vi "pruebas.vi"(11 "Image":T1) -> ()   [LabVIEW 2020]
uses:
  <vilib>/vision/Image Controls.llb/IMAQ Image.ctl
  <vilib>/picture/picture.llb/Draw True-Color Pixmap.vi
  <vilib>/Analysis/NI_AALBase.lvlib
panel:
  in  "alfa":dbl(slide) scale=0.0..5.0
  in  "S":dbl=30.0 format="%#_13g"
  in  "V":dbl=20.0 format="%#_13g"
  in  "Tamaño de máscara":i32
  out "Color":u32(colorbox)
  out "2D Picture":picture
  in  "Factor diezmado":i32=60
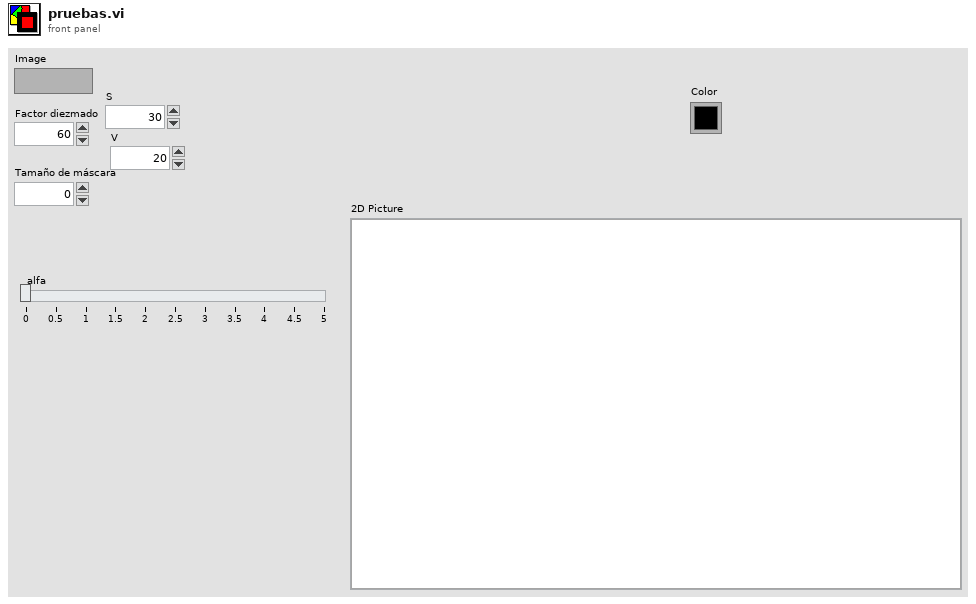
[diagram p1: front panel]
types:
  T1 = typedef "IMAQ Image.ctl" = refnum<image>
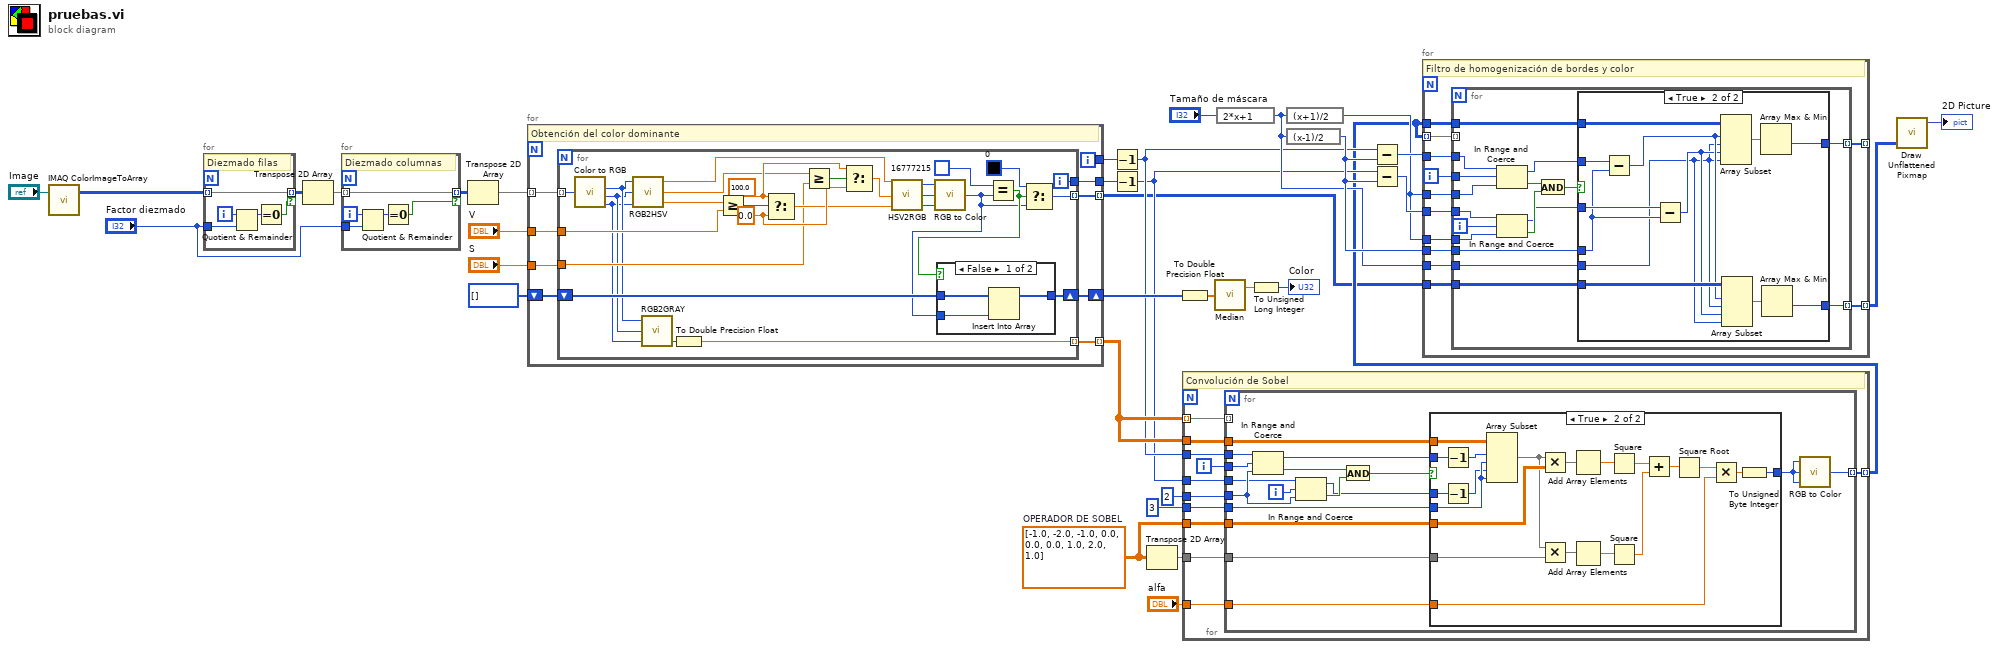
[diagram p0: block diagram]
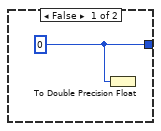
[diagram p2: hidden frame]
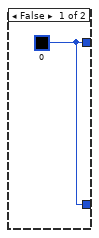
[diagram p3: hidden frame]
diagram:
  w5 = dbl[][] [[-1.0, -2.0, -1.0], [0.0, 0.0, 0.0], [1.0, 2.0, 1.0]]  # OPERADOR DE SOBEL
  n1 = call "IMAQ ColorImageToArray"("Image"="Image") -> ("Image Pixels (U32)"=w31:u32[][])  [unwired: 3 in, 2 out]
  n2 = for {
    tunnel: w31 -> [w39] mode=indexing
    tunnel: [w39] -> w34 mode=indexing if=w36
    tunnel: "Factor diezmado" -> [w35]
    i -> [w38]
    # "Diezmado filas"
    n3 = Quotient & Remainder(x=w38, y=w35) -> (x-y*floor(x/y)=w37:i32)  [unwired: 1 out]
    n4 = Equal To 0?(x=w37) -> (x = 0?=w36:bool)
  }
  n5 = Transpose 2D Array(2D array=w34) -> (transposed array=w33:u32[][])
  n6 = for {
    tunnel: w33 -> [w44] mode=indexing
    tunnel: [w44] -> w30 mode=indexing if=w41
    tunnel: "Factor diezmado" -> [w40]
    i -> [w43]
    # "Diezmado columnas"
    n7 = Quotient & Remainder(x=w43, y=w40) -> (x-y*floor(x/y)=w42:i32)  [unwired: 1 out]
    n8 = Equal To 0?(x=w42) -> (x = 0?=w41:bool)
  }
  n9 = Transpose 2D Array(2D array=w30) -> (transposed array=w27:u32[][])
  n10 = for {
    tunnel: w27 -> [w53] mode=indexing
    tunnel: [w52] -> w2 mode=indexing
    tunnel: [w51] -> w24
    tunnel: [w50] -> w25
    tunnel: "V" -> [w49]
    tunnel: "S" -> [w48]
    shift-right: [w46] -> w16
    shift-left: u32[] [] -> [w47]
    tunnel: [w45] -> w11 mode=indexing
    i -> [w50]
    # "Obtención del color dominante"
    n11 = for {
      tunnel: w53 -> [w59] mode=indexing
      tunnel: [w69] -> w52 mode=indexing
      tunnel: [w68] -> w51
      tunnel: w49 -> [w67]
      tunnel: w48 -> [w66]
      shift-right: [w64] -> w46
      shift-left: w47 -> [w65]
      tunnel: [w54] -> w45 mode=indexing
      i -> [w68]
      w78 = 0.0 ("f")
      w79 = 100.0 ("t")
      n12 = call <vilib>:"Color to RGB.vi"("Color"=w59) -> ("R"=w58:u8, "G"=w57:u8, "B"=w56:u8)  [unwired: 1 out]
      n13 = call "RGB2HSV.vi"("B"=w56, "G"=w57, "R"=w58) -> ("V"=w60:dbl, "S"=w61:dbl, "H"=w75:dbl)
      n14 = call "RGB2GRAY.vi"("B"=w56, "G"=w57, "R"=w58) -> ("gray B"=w55:u8)  [unwired: 2 out]
      n15 = To Double Precision Float(number=w55) -> (double precision float=w54:dbl)
      n16 = Greater Or Equal?(x=w60, y=w67) -> (x >= y?=w81:bool)
      n17 = Select(t=w79, s=w81, f=w78) -> (s? t:f=w77:dbl)
      n18 = Greater Or Equal?(x=w61, y=w66) -> (x >= y?=w80:bool)
      n19 = Select(t=w79, s=w80, f=w78) -> (s? t:f=w76:dbl)
      n20 = call "HSV2RGB.vi"("V"=w77, "S"=w76, "H"=w75) -> ("B"=w72:u8, "G"=w73:u8, "R"=w74:u8)
      n21 = call <vilib>:"RGB to Color.vi"("B"=w72, "G"=w73, "R"=w74) -> ("Color"=w62:u32)
      n22 = Equal?(x=u32 16777215, y=w62) -> (x = y?=w63:bool)
      n23 = case shown="False" w63 {
        tunnel: w65 -> [w84 w85]
        tunnel: [w83 w85] -> w64
        tunnel: w62 -> [w82 _]
        frame False {
          n24 = Insert Into Array(array=w84, new element=w82) -> (w83:u32[])  [unwired: 1 in]
        }
        frame True {
        }
      }
      n25 = Select(t=u32 0, s=w63, f=w62) -> (s? t:f=w69:u32)
    }
  }
  n26 = Decrement(x=w25) -> (x-1=w10:i32)
  n27 = Decrement(x=w24) -> (x-1=w9:i32)
  n28 = Transpose 2D Array(2D array=w5) -> (transposed array=w6:dbl[][])
  n29 = To Double Precision Float(number=w16) -> (double precision float=w12:dbl[])
  n30 = for {
    tunnel: w11 -> [w95] mode=indexing
    tunnel: w11 -> [w96]
    tunnel: w10 -> [w94]
    tunnel: w9 -> [w92]
    tunnel: [w91] -> w3 mode=indexing
    tunnel: 2 -> [w90]
    tunnel: 3 -> [w89]
    tunnel: w5 -> [w88]
    tunnel: w6 -> [w87]
    tunnel: "alfa" -> [w86]
    i -> [w93]
    # "Convolución de Sobel"
    n31 = for {
      tunnel: w96 -> [w105]
      tunnel: w94 -> [w113]
      tunnel: w92 -> [w111]
      tunnel: w90 -> [w112]
      tunnel: w89 -> [w102]
      tunnel: w93 -> [w110]
      tunnel: w88 -> [w101]
      tunnel: [w98] -> w91 mode=indexing
      tunnel: w95 -> [_] mode=indexing
      tunnel: w87 -> [w100]
      tunnel: w86 -> [w99]
      i -> [w109]
      n32 = In Range and Coerce(upper limit=w113, x=w110, lower limit=w112) -> (coerced(x)=w104:i32, In Range?=w108:bool)
      n33 = In Range and Coerce(upper limit=w111, x=w109, lower limit=w112) -> (coerced(x)=w103:i32, In Range?=w107:bool)
      n34 = And(x=w108, y=w107) -> (x .and. y?=w106:bool)
      n35 = case shown="True" w106 {
        tunnel: w105 -> [_ w132]
        tunnel: w104 -> [_ w134]
        tunnel: w103 -> [_ w133]
        tunnel: w102 -> [_ w130]
        tunnel: w101 -> [_ w128]
        tunnel: [w114 w116] -> w97
        tunnel: w100 -> [_ w126]
        tunnel: w99 -> [_ w117]
        frame False {
          w114 = u8 0
          n36 = To Double Precision Float(number=w114) -> ()  [unwired: 1 out]
        }
        frame True {
          n37 = Decrement(x=w134) -> (x-1=w131:i32)
          n38 = Decrement(x=w133) -> (x-1=w129:i32)
          n39 = Array Subset(array=w132, index (row)=w131, length (row)=w130, index (col)=w129, length (col)=w130) -> (w125:dbl[][])
          n40 = Multiply(x=w125, y=w128) -> (x*y=w127:dbl[][])
          n41 = Multiply(x=w125, y=w126) -> (x*y=w124:dbl[][])
          n42 = Add Array Elements(numeric array=w127) -> (sum=w123:dbl)
          n43 = Add Array Elements(numeric array=w124) -> (sum=w122:dbl)
          n44 = Square(x=w123) -> (x^2=w121:dbl)
          n45 = Square(x=w122) -> (x^2=w120:dbl)
          n46 = Add(x=w121, y=w120) -> (x+y=w119:dbl)
          n47 = Square Root(x=w119) -> (sqrt(x)=w118:dbl)
          n48 = Multiply(x=w118, y=w117) -> (x*y=w115:dbl)
          n49 = To Unsigned Byte Integer(number=w115) -> (unsigned 8bit integer=w116:u8)
        }
      }
      n50 = call <vilib>:"RGB to Color.vi"("B"=w97, "G"=w97, "R"=w97) -> ("Color"=w98:u32)
    }
  }
  n51 = call <vilib>:"Median.vi"("X"=w12) -> ("median"=w15:dbl)  [unwired: 1 out]
  n52 = expression code="2*x+1"("Tamaño de máscara") -> (w14:i32)
  n53 = To Unsigned Long Integer(number=w15) -> (unsigned 32bit integer=→"Color":u32)
  n54 = expression code="(x+1)/2"(w14) -> (w21:i32)
  n55 = expression code="(x-1)/2"(w14) -> (w20:i32)
  n56 = Subtract(x=w10, y=w20) -> (x-y=w23:i32)
  n57 = Subtract(x=w9, y=w20) -> (x-y=w22:i32)
  n58 = for {
    tunnel: w3 -> [w145] mode=indexing
    tunnel: w21 -> [w144]
    tunnel: w23 -> [w143]
    tunnel: w21 -> [w142]
    tunnel: w22 -> [w141]
    tunnel: w3 -> [w140]
    tunnel: w20 -> [w139]
    tunnel: w14 -> [w138]
    tunnel: [w137] -> _ mode=indexing
    tunnel: w2 -> [w136]
    tunnel: [w135] -> w1 mode=indexing
    i -> [w146]
    # "Filtro de homogenización de bordes y color"
    n59 = for {
      tunnel: w146 -> [w155]
      tunnel: w145 -> [_] mode=indexing
      tunnel: w144 -> [w163]
      tunnel: w143 -> [w162]
      tunnel: w142 -> [w160]
      tunnel: w141 -> [w152]
      tunnel: w140 -> [w156]
      tunnel: w139 -> [w154]
      tunnel: w138 -> [w153]
      tunnel: [w151] -> w137 mode=indexing
      tunnel: w136 -> [w148]
      tunnel: [w147] -> w135 mode=indexing
      i -> [w161]
      n60 = In Range and Coerce(upper limit=w162, x=w155, lower limit=w163) -> (coerced(x)=w150:i32, In Range?=w159:bool)
      n61 = In Range and Coerce(upper limit=w152, x=w161, lower limit=w160) -> (coerced(x)=w149:i32, In Range?=w158:bool)
      n62 = And(x=w159, y=w158) -> (x .and. y?=w157:bool)
      n63 = case shown="True" w157 {
        tunnel: w156 -> [_ w176]
        tunnel: w150 -> [_ w175]
        tunnel: w154 -> [_ w173]
        tunnel: w153 -> [_ w165]
        tunnel: w149 -> [_ w174]
        tunnel: [w164 w171] -> w151
        tunnel: w148 -> [_ w169]
        tunnel: [w164 w168] -> w147
        frame False {
          w164 = u32 0
        }
        frame True {
          n64 = Subtract(x=w175, y=w173) -> (x-y=w167:i32)
          n65 = Subtract(x=w174, y=w173) -> (x-y=w166:i32)
          n66 = Array Subset(array=w176, index (row)=w167, length (row)=w165, index (col)=w166, length (col)=w165) -> (w172:u32[][])
          n67 = Array Subset(array=w169, index (row)=w167, length (row)=w165, index (col)=w166, length (col)=w165) -> (w170:u32[][])
          n68 = Array Max & Min(array=w172) -> (min value=w171:u32)  [unwired: 3 out]
          n69 = Array Max & Min(array=w170) -> (min value=w168:u32)  [unwired: 3 out]
        }
      }
    }
  }
  n70 = call-poly <vilib>:"Draw Unflattened Pixmap.vi"("data (RGB format)"=w1) -> ("new picture"=→"2D Picture":picture)  [unwired: 8 in]
